vi "STD_DO浓度算法.vi"(8 "溶解氧饱和度值":dbl, 9 "水温":dbl, 10 "大气压补偿":dbl=101.35, 11 "盐度补偿":dbl) -> (3 "DataDo_mgL":dbl)   [LabVIEW 2016, in "斯坦道多参数.lvlib"]
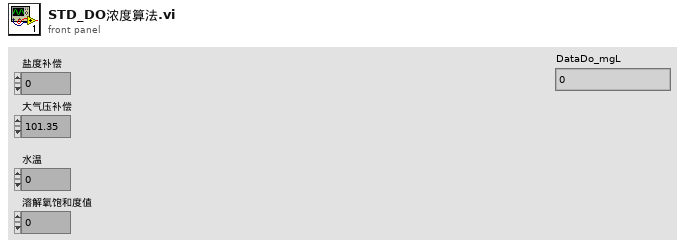
[diagram p1: front panel]
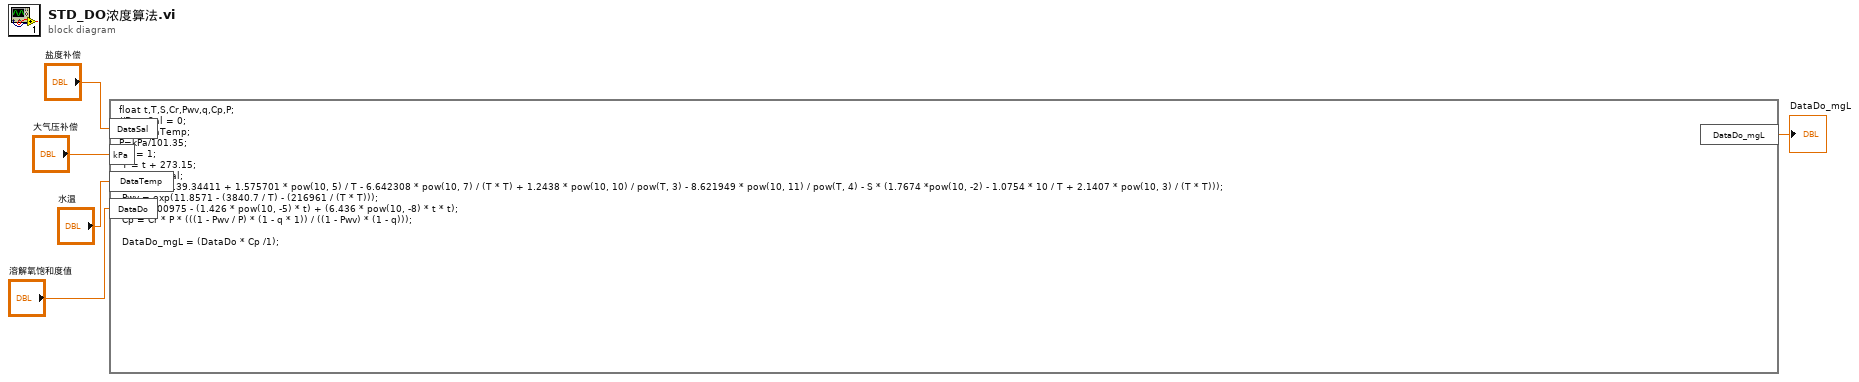
[diagram p0: block diagram]
diagram:
  n1 = formula code="float t,T,S,Cr,Pwv,q,Cp,P;\n//DataSal = 0; \nt = DataTemp;\nP=kPa/101.35;\n //P = 1;\n T = t + 273.15;\n S = DataSal;\n Cr = exp(-139.34411 + 1.575701 * pow(10, 5) / T - 6.642308 * pow(10, 7) / (T * T) + 1.2438 * pow(10, 10) / pow(T, 3) - 8.621949 * pow(10, 11) / pow(T, 4) - S * (1.7674 *pow(10, -2) - 1.0754 * 10 / T + 2.1407 * pow(10, 3) / (T * T)));\n Pwv = exp(11.8571 - (3840.7 / T) - (216961 / (T * T)));\n q = 0.000975 - (1.426 * pow(10, -5) * t) + (6.436 * pow(10, -8) * t * t);\n Cp = Cr * P * (((1 - Pwv / P) * (1 - q * 1)) / ((1 - Pwv) * (1 - q)));\n\n DataDo_mgL = (DataDo * Cp /1);" ("公式节点")("DataTemp"="水温", "DataDo"="溶解氧饱和度值", "DataSal"="盐度补偿", "kPa"="大气压补偿") -> ("DataDo_mgL"=→"DataDo_mgL":dbl)
